vi "PredetControlSequence (SubVI).vi"(8 "Stop Button":bool) -> (11 "PredetState":T1)   [LabVIEW 2016]
uses:
  PredetControl.ctl
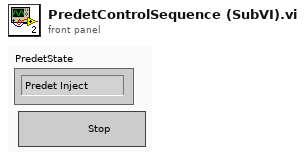
[diagram p1: front panel]
types:
  T1 = typedef "PredetControl.ctl" = enum16{"Predet Inject", "Predet Fire", "Stop"}
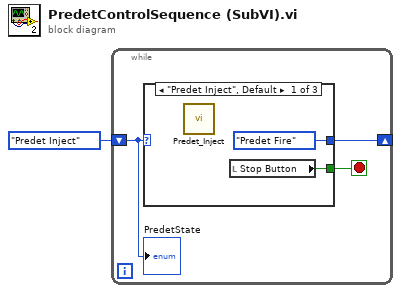
[diagram p0: block diagram]
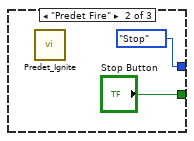
[diagram p2: hidden frame]
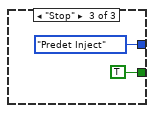
[diagram p3: hidden frame]
diagram:
  n1 = while {
    shift-right: [w3] -> _
    shift-left: PredetControl."Predet Inject" -> [w4]
    stop <- w2 stop-if-true
    n2 = case shown="\"Predet Inject\", Default" w4 {
      tunnel: [PredetControl."Predet Fire" PredetControl."Stop" PredetControl."Predet Inject"] -> w3
      tunnel: [w5 "Stop Button" TRUE] -> w2
      frame "Predet Inject", Default {
        n3 = call "Predet_Inject.vi"() -> ()  [unwired: 12 in]
        n4 = local read "Stop Button"() -> (w5:bool)
      }
      frame "Predet Fire" {
        n5 = call "Predet_Ignite.vi"() -> ()  [unwired: 10 in, 2 out]
      }
      frame "Stop" {
      }
    }
    "PredetState" <- w4
  }
